vi "Filter Keywords Based on Regular Expression.vi"(8 "error in (no error)":errorcluster, 10 "Regular Expression":string, 11 "Words":string[](array[string])) -> (0 "error out":errorcluster, 3 "Filters Words":string[](array[string]))   [LabVIEW 2013]
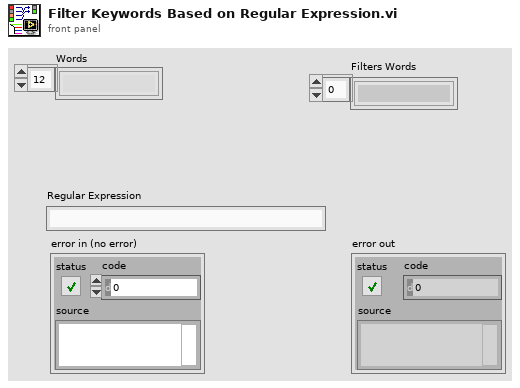
[diagram p1: front panel]
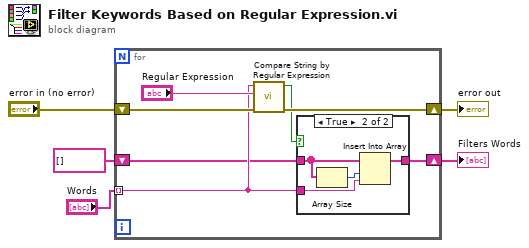
[diagram p0: block diagram]
diagram:
  n1 = for {
    tunnel: "Words" -> [w8] mode=indexing
    shift-right: [w11] -> w4
    shift-left: "error in (no error)" -> [w12]
    shift-right: [w6] -> w5
    shift-left: string[] [] -> [w7]
    n2 = call "Compare String by Regular Expression.vi"("error in"=w12, "regular expression"="Regular Expression", "String"=w8) -> ("error out"=w11:errorcluster, "x = y?"=w9:bool)  [unwired: 7 in]
    n3 = case shown="True" w9 {
      tunnel: w8 -> [_ w17]
      tunnel: w7 -> [w13 w15]
      tunnel: [w13 w14] -> w6
      frame False {
      }
      frame True {
        n4 = Array Size(array=w15) -> (size(s)=w16:i32)
        n5 = Insert Into Array(array=w15, index=w16, new element=w17) -> (w14:string[])
      }
    }
  }
  "Filters Words" <- w5
  "error out" <- w4
